vi "Read Execute_.vi"(8 "error in (no error)":errorcluster, 11 "Beep Msg in":refnum<class "Beep Msg.lvclass">) -> (0 "error out":errorcluster, 2 "Execute?":bool=TRUE, 3 "Beep Msg out":refnum<class "Beep Msg.lvclass">)   [LabVIEW 2016, in "CS++BeepActor.lvlib" / "Beep Msg.lvclass"]
uses:
  Beep Msg.lvclass
  Beep Msg.lvclass/Beep Msg.ctl
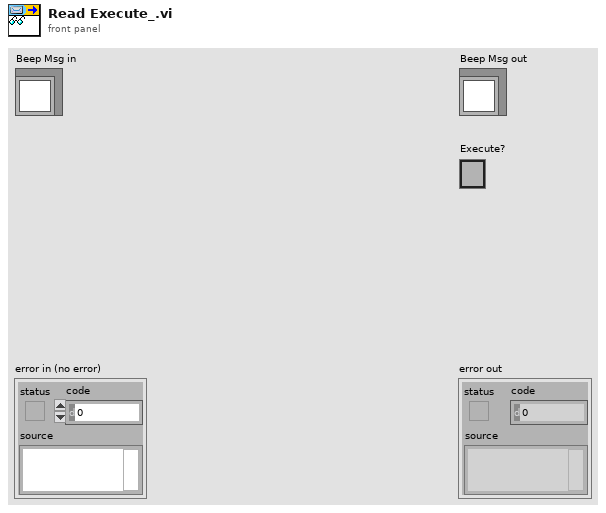
[diagram p1: front panel]
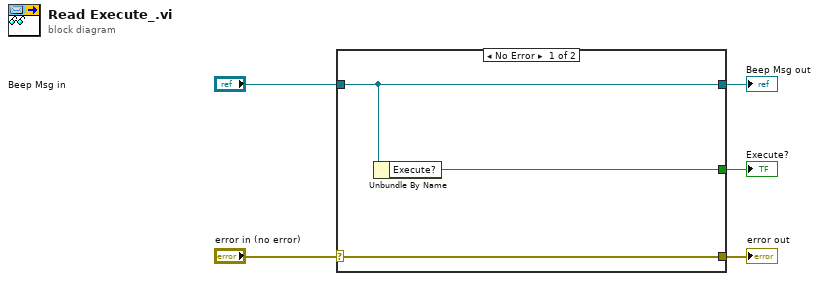
[diagram p0: block diagram]
diagram:
  n1 = case shown="No Error" "error in (no error)" {
    selector: "error in (no error)" -> [w8 w9]
    tunnel: [w8 w9] -> w4
    tunnel: [w7 w10] -> w2
    tunnel: "Beep Msg in" -> [w7 w10]
    tunnel: [w6 _] -> w1
    frame No Error {
      n2 = Unbundle By Name(w7) -> ("Execute?"=w6:bool)
    }
    frame Error {
    }
  }
  "error out" <- w4
  "Beep Msg out" <- w2
  "Execute?" <- w1
